vi "Fitness Tracker - Main.vi"() -> ()   [LabVIEW 2021]
uses:
  Lab 5/Lab 5 Code/Heading_TDef.ctl
  Main - States_SubVI.ctl
  <vilib>/Platform/TimedLoop/XDataNode/timing_clust.ctl
  <vilib>/Platform/TimedLoop/XDataNode/nitl_modes.ctl
  <vilib>/Platform/TimedLoop/XDataNode/wakeup.ctl
  ProducerConsumer Data Cluster_TDef.ctl
  Measurement Data Cluster_TDef.ctl
  <vilib>/myRIO/Instrument Drivers/Onboard IO/I2C/typedefs/I2C User Configuration.ctl
  <vilib>/myRIO/Instrument Drivers/Onboard IO/I2C/typedefs/I2C Transfer Rate.ctl
  <vilib>/myRIO/Instrument Drivers/Onboard IO/I2C/typedefs/I2C Reference.ctl
  <vilib>/myRIO/Common/Instrument Driver Framework/Utilities/typedefs/myRIO Generic Hardware Reference.ctl
  <vilib>/myRIO/Common/Instrument Driver Framework/Utilities/typedefs/Hardware Version Enum.ctl
  <vilib>/myRIO/Common/Instrument Driver Framework/Utilities/typedefs/myRIO v1.0 Reference.ctl
  <vilib>/myRIO/Common/Instrument Driver Framework/Utilities/typedefs/Generic FPGA Reference.ctl
  <vilib>/myRIO/Common/Instrument Driver Framework/myRIO v1.0/I2C/typedefs/I2C Channels Enum.ctl
  <vilib>/myRIO/Instrument Drivers/Onboard IO/I2C/typedefs/I2C Configuration.ctl
  <vilib>/userDefined/High Color/nirio_resource_hc.ctl
  <vilib>/myRIO/Common/Instrument Driver Framework/Utilities/vis/Is FPGA Ref Available.vi
  <vilib>/myRIO/Common/Instrument Driver Framework/myRIO v1.0/I2C/vis/myRIO v1.1 Open I2C.vi
  <vilib>/myRIO/Instrument Drivers/Onboard IO/I2C/vis/Configure.vi
  <vilib>/myRIO/Common/Instrument Driver Framework/Utilities/vis/Validate Channels.vi
  <vilib>/myRIO/Common/Instrument Driver Framework/myRIO v1.0/I2C/vis/myRIO v1.0 Reserve I2C.vi
  <vilib>/myRIO/Common/Instrument Driver Framework/myRIO v1.0/I2C/vis/myRIO v1.0 Build MUX Configuration I2C.vi
  <vilib>/myRIO/Common/Instrument Driver Framework/myRIO v1.0/Resource Manager/vis/myRIO v1.0 Reserve Channel List.vi
  <vilib>/myRIO/Common/Instrument Driver Framework/myRIO v1.0/Resource Manager/vis/myRIO v1.0 Create Configuration List.vi
  <vilib>/myRIO/Common/Instrument Driver Framework/myRIO v1.0/Resource Manager/vis/myRIO v1.0 Reserve Channel.vi
  <vilib>/myRIO/Common/Instrument Driver Framework/myRIO v1.0/Resource Manager/vis/myRIO v1.0 Unreserve Channel.vi
  <vilib>/myRIO/Common/Instrument Driver Framework/myRIO v1.0/Resource Manager/vis/myRIO v1.0 Build Mutex Name.vi
  <vilib>/Utility/error.llb/Error Cluster From Error Code.vi
  <vilib>/myRIO/Common/Instrument Driver Framework/myRIO v1.0/DIO/vis/myRIO v1.0 Write DIO.vi
  <vilib>/Utility/VariantDataType/GetNumericInfo.vi
  <vilib>/myRIO/Common/Instrument Driver Framework/myRIO v1.0/myRIO v1.1 Open.vi
  <vilib>/myRIO/Common/Instrument Driver Framework/Utilities/vis/IO Manager.vi
  <vilib>/myRIO/Common/Instrument Driver Framework/Utilities/vis/Configuration Manager.vi
  <vilib>/myRIO/Common/Instrument Driver Framework/myRIO v1.0/Resource Manager/vis/myRIO v1.0 Configure IO.vi
  <vilib>/myRIO/Common/Instrument Driver Framework/myRIO v1.0/myRIO v1.0 Close.vi
  <vilib>/myRIO/Common/Instrument Driver Framework/myRIO v1.0/I2C/vis/myRIO v1.0 Configure I2C.vi
  <vilib>/myRIO/Common/Instrument Driver Framework/myRIO v1.0/I2C/vis/myRIO v1.0 Write I2C.vi
  <vilib>/platform/TimedLoop/XDataNode/XDataNode.xnode
  <vilib>/myRIO/Express VI/Onboard IO/I2C/I2C Express VI.xnode
  <vilib>/myRIO/Instrument Drivers/Onboard IO/I2C/vis/myRIO I2C Open.xnode
  <vilib>/Platform/TimedLoop/XDataNode/XDNodeRunTimeDep.lvlib
  <vilib>/myRIO/Instrument Drivers/Onboard IO/DIO/DIO.lvlib
  <vilib>/myRIO/Instrument Drivers/Onboard IO/AI/AI.lvlib
  <vilib>/myRIO/Instrument Drivers/Onboard IO/I2C/I2C.lvlib
panel:
  out "x > y?":bool
  out "Gyro Rotation Out (degrees)":dbl[](array[numeric])
  out "element":dbl
  out "error out 4":errorcluster
  in  "error in (no error) 2":errorcluster
  out "error out 3":errorcluster
  out "Loop 2 Time":i32
  out "GNRMC String Array":string[](array[string])
  out "Step Counter Map":T1(graph)
  out "Producer Loop Time (ms)":i32
  out "Consumer Loop Time (ms)":i32
  out "Heart Rate":dbl
  out "Latitude N (deg)":dbl
  out "DIP State":T2
  out "Time Elapsed (min)":dbl
  out "error out 2":errorcluster caption="error out"
  out "North":dbl
  out "East":dbl
  out "Heading String 2":T3
  out "Heading":dbl
  out "Steps":i32
  in  "error in (no error)":errorcluster
  in  "Reset Gyro":bool
  out "Acceleration (g)":T4(graph)
  out "Velocity":T5(graph)
  out "Rotation":T4(graph)
  out "Acceleration (ms^2)":dbl[](array[numeric])
  out "Velocity Cluster Out":cluster{i16, i16, i16}
  out "Rotation Cluster Out":T6
  out "error out":errorcluster
  in  "stop":bool
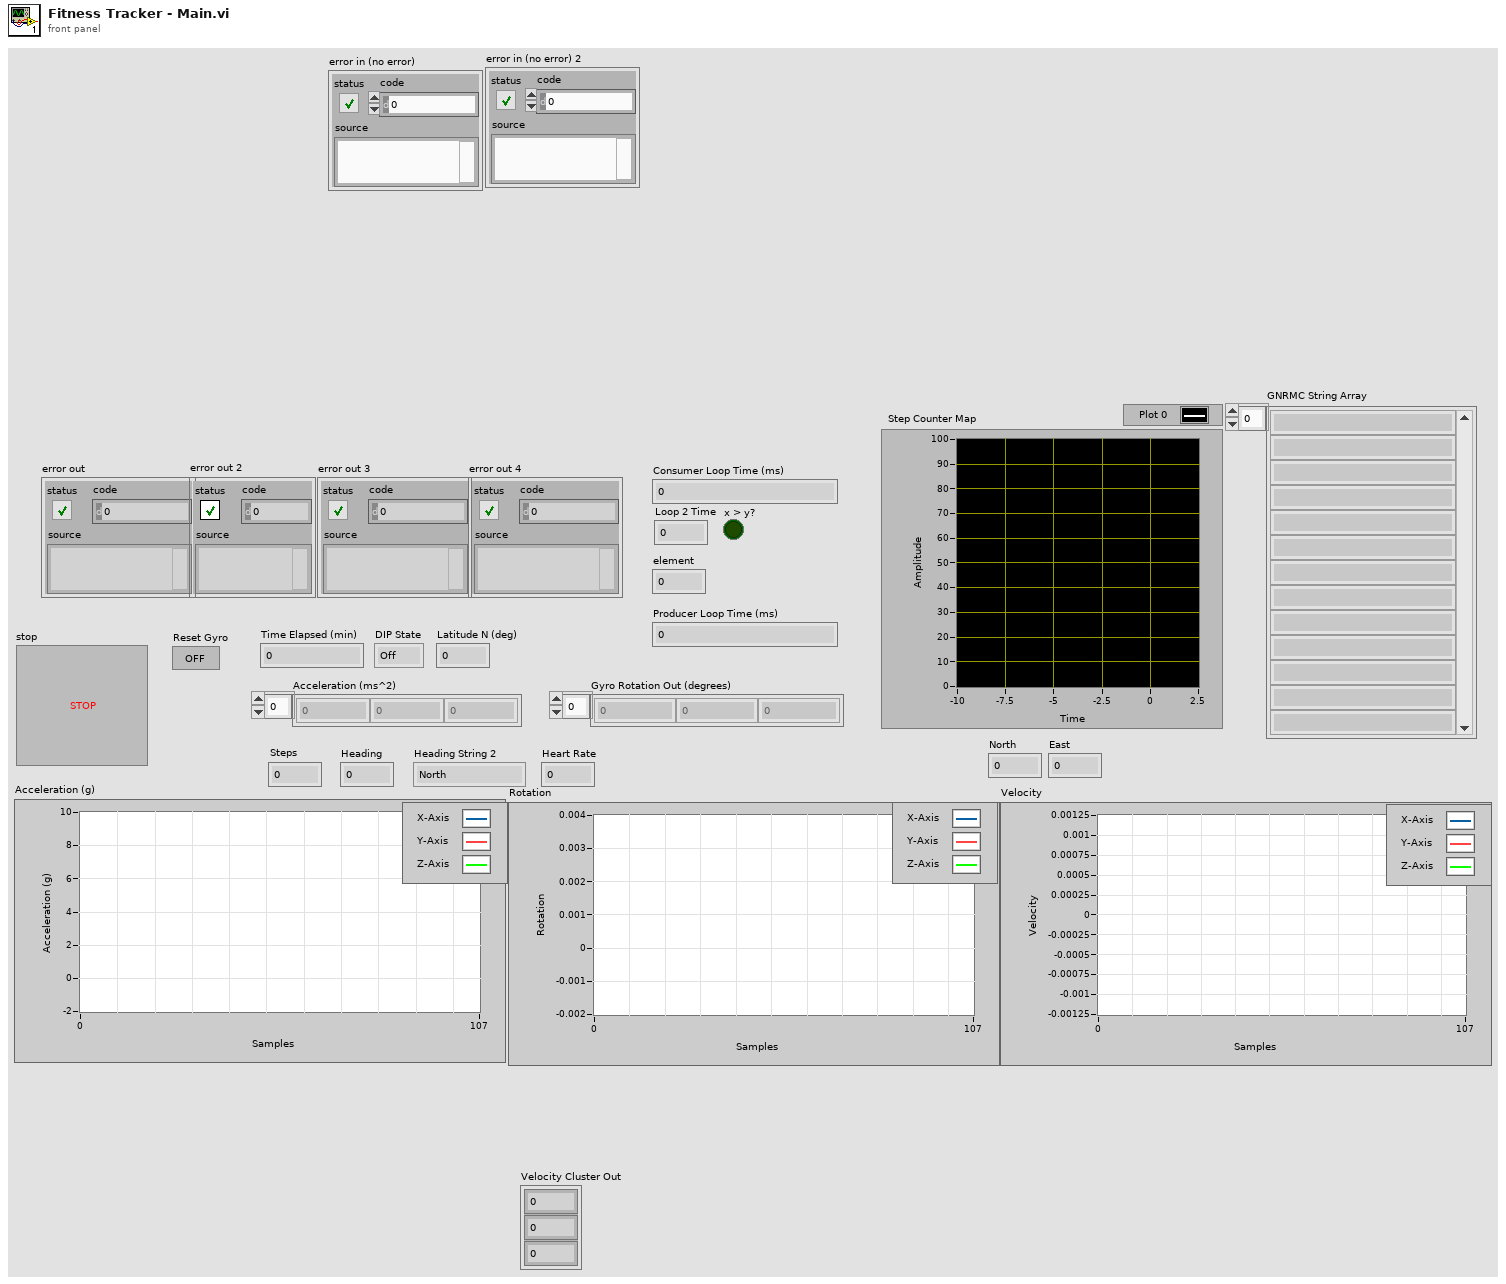
[diagram p1: front panel]
types:
  T1 = cluster{"X Displacement Array ":dbl[], "Y Displacement Array ":dbl[]}
  T2 = typedef "Main - States_SubVI.ctl" = enum16{"Off", "Record", "Upload", "Shutdown", "Error"}
  T3 = typedef "Heading_TDef.ctl" = enum16{"North ", "North East", "East", "Southeast", "South", "Southwest", "West", "Northwest"}
  T4 = cluster{"X-Axis":dbl, "Y-Axis":dbl, "Z-Axis":dbl}
  T5 = cluster{"Velocity":dbl, "Velocity":dbl, "Velocity":dbl}
  T6 = cluster{"integral x(t)":dbl, "integral x(t)":dbl, "integral x(t)":dbl}
  T7 = typedef "Measurement Data Cluster_TDef.ctl" = cluster{"Step Count":i32, "East Displacement":dbl, "North Displacement":dbl, "Longitude":dbl, "Latitude":dbl, "Heart Rate":dbl, "Time Elapsed (min)":dbl}
  T8 = typedef "ProducerConsumer Data Cluster_TDef.ctl" = cluster{"Accelerometer":dbl[], "Gyro":dbl[], "Magnetometer":dbl, "Time":i32, "Pulse":dbl}
  T9 = typedef "DIO.lvlib/DIO Reference.ctl" = cluster{"myRIO Reference":T10, "DIO Channels List":T14}
  T10 = typedef "myRIO Generic Hardware Reference.ctl" = cluster{"myRIO Model":T11, "myRIO Hardware Reference":T12}
  T11 = typedef "Hardware Version Enum.ctl" = enum16{"Unknown", "myRIO-1900", "myRIO-1950", "roboRIO", "NI ELVIS RIO CM", "ELVIS III"}
  T12 = typedef "myRIO v1.0 Reference.ctl" = cluster{"Generic FPGA Reference":T13, "Allow multiple opens":bool}
  T13 = typedef "Generic FPGA Reference.ctl" = refnum<k20>
  T14 = typedef "DIO Channels List.ctl" = T15[]
  T15 = typedef "DIO Channels Enum.ctl" = enum16{"Not Connected", "C/DIO0", "C/DIO1", "C/DIO2", "C/DIO3", "C/DIO4", "C/DIO5", "C/DIO6", "C/DIO7", "A/DIO0", "A/DIO1", "A/DIO2", "A/DIO3", "A/DIO4", "A/DIO5", "A/DIO6", "A/DIO7", "A/DIO8", "A/DIO9", "A/DIO10", "A/DIO11", "A/DIO12", "A/DIO13", "A/DIO14", "A/DIO15", "A/DIO16", "A/DIO17", "A/DIO18", "A/DIO19", "B/DIO0", "B/DIO1", "B/DIO2", "B/DIO3", "B/DIO4", "B/DIO5", "B/DIO6", "B/DIO7", "B/DIO8", "B/DIO9", "B/DIO10", "B/DIO11", "B/DIO12", "B/DIO13", "B/DIO14", "B/DIO15", "B/DIO16", "B/DIO17", "B/DIO18", "B/DIO19", "LED0", "LED1", "LED2", "LED3", "Button0", "DIO/DIO0", "DIO/DIO1", "DIO/DIO2", "DIO/DIO3", "DIO/DIO4", "DIO/DIO5", "DIO/DIO6", "DIO/DIO7", "DIO/DIO8", "DIO/DIO9", "SPI/CS0", "SPI/CS1", "SPI/CS2", "SPI/CS3", "LED RADIO (Green)", "LED RADIO (Red)", "LED COMM (Green)", "LED COMM (Red)", "LED MODE (Green)", "LED MODE (Red)"}
  T16 = typedef "XDNodeRunTimeDep.lvlib/timing_clust.ctl" = cluster{"Expected End [f-1]":u64, "Actual End [f-1]":u64, "Finished Late? [f-1]":bool, "Expected End [i-1]":u64, "Actual End [i-1]":u64, "Finished Late? [i-1]":bool, "Expected Start [i]":u64, "Actual Start [i]":u64, "Expected Start [f]":u64, "Actual Start [f]":u64, "Source Name":string, "Structure Name":string, "Period":i64, "Deadline":i64, "Offset":i64, "Start":i64, "Priority":i32, "Timeout":i32, "Mode":T17, "Wakeup Reason":T18, "Error":errorcluster, "Source Type":string, "Secondary Source Type":string, "Global End Time":u64, "Global Start Time":u64, "Frame Duration":u64, "Iteration Duration":u64, "Assigned CPU":i32, "I/O Scan Engine Mode":u32}
  T17 = typedef "XDNodeRunTimeDep.lvlib/nitl_modes.ctl" = enum32{"No Change", "Process missed periods, maintain original phase", "Discard missed periods, maintain original phase", "Process missed periods, ignore original phase", "Discard missed periods, ignore original phase"}
  T18 = typedef "XDNodeRunTimeDep.lvlib/wakeup.ctl" = enum32{"Normal", "Aborted", "Asynchronous wakeup", "Timing source error", "Timed loop error", "Timeout"}
  T19 = typedef "I2C.lvlib/I2C Reference.ctl" = cluster{"myRIO Reference":T10, "I2C Channels Enum":T20, "I2C Configuration":T21}
  T20 = typedef "I2C Channels Enum.ctl" = enum16{"Not Connected", "A/I2C", "B/I2C", "I2C/I2C"}
  T21 = typedef "I2C.lvlib/I2C Configuration.ctl" = cluster{"I2C Transfer Rate":T22}
  T22 = typedef "I2C.lvlib/I2C Transfer Rate.ctl" = enum16{"Standard mode (100 kbps)", "Fast mode (400 kbps)"}
  T23 = typedef "AI.lvlib/AI Reference.ctl" = cluster{"myRIO Reference":T10, "AI Channels List":T24, "AI Scaling Constants List":T26}
  T24 = typedef "AI Channels List.ctl" = T25[]
  T25 = typedef "AI Channels Enum.ctl" = enum16{"Not Connected", "AudioIn/Left", "AudioIn/Right", "C/AI0", "C/AI1", "A/AI0", "A/AI1", "A/AI2", "A/AI3", "A/AI4", "A/AI5", "A/AI6", "A/AI7", "B/AI0", "B/AI1", "B/AI2", "B/AI3", "B/AI4", "B/AI5", "B/AI6", "B/AI7", "AI/AI0", "AI/AI1", "AI/AI2", "AI/AI3", "A/AI0 (DIFF)", "A/AI1 (DIFF)", "A/AI2 (DIFF)", "A/AI3 (DIFF)", "B/AI0 (DIFF)", "B/AI1 (DIFF)", "B/AI2 (DIFF)", "B/AI3 (DIFF)"}
  T26 = typedef "Analog Scaling Constants List.ctl" = T27[]
  T27 = typedef "Analog Scaling Constants.ctl" = cluster{"LSB Weight (Volts)":dbl, "Offset (Volts)":dbl, "Signed?":bool}
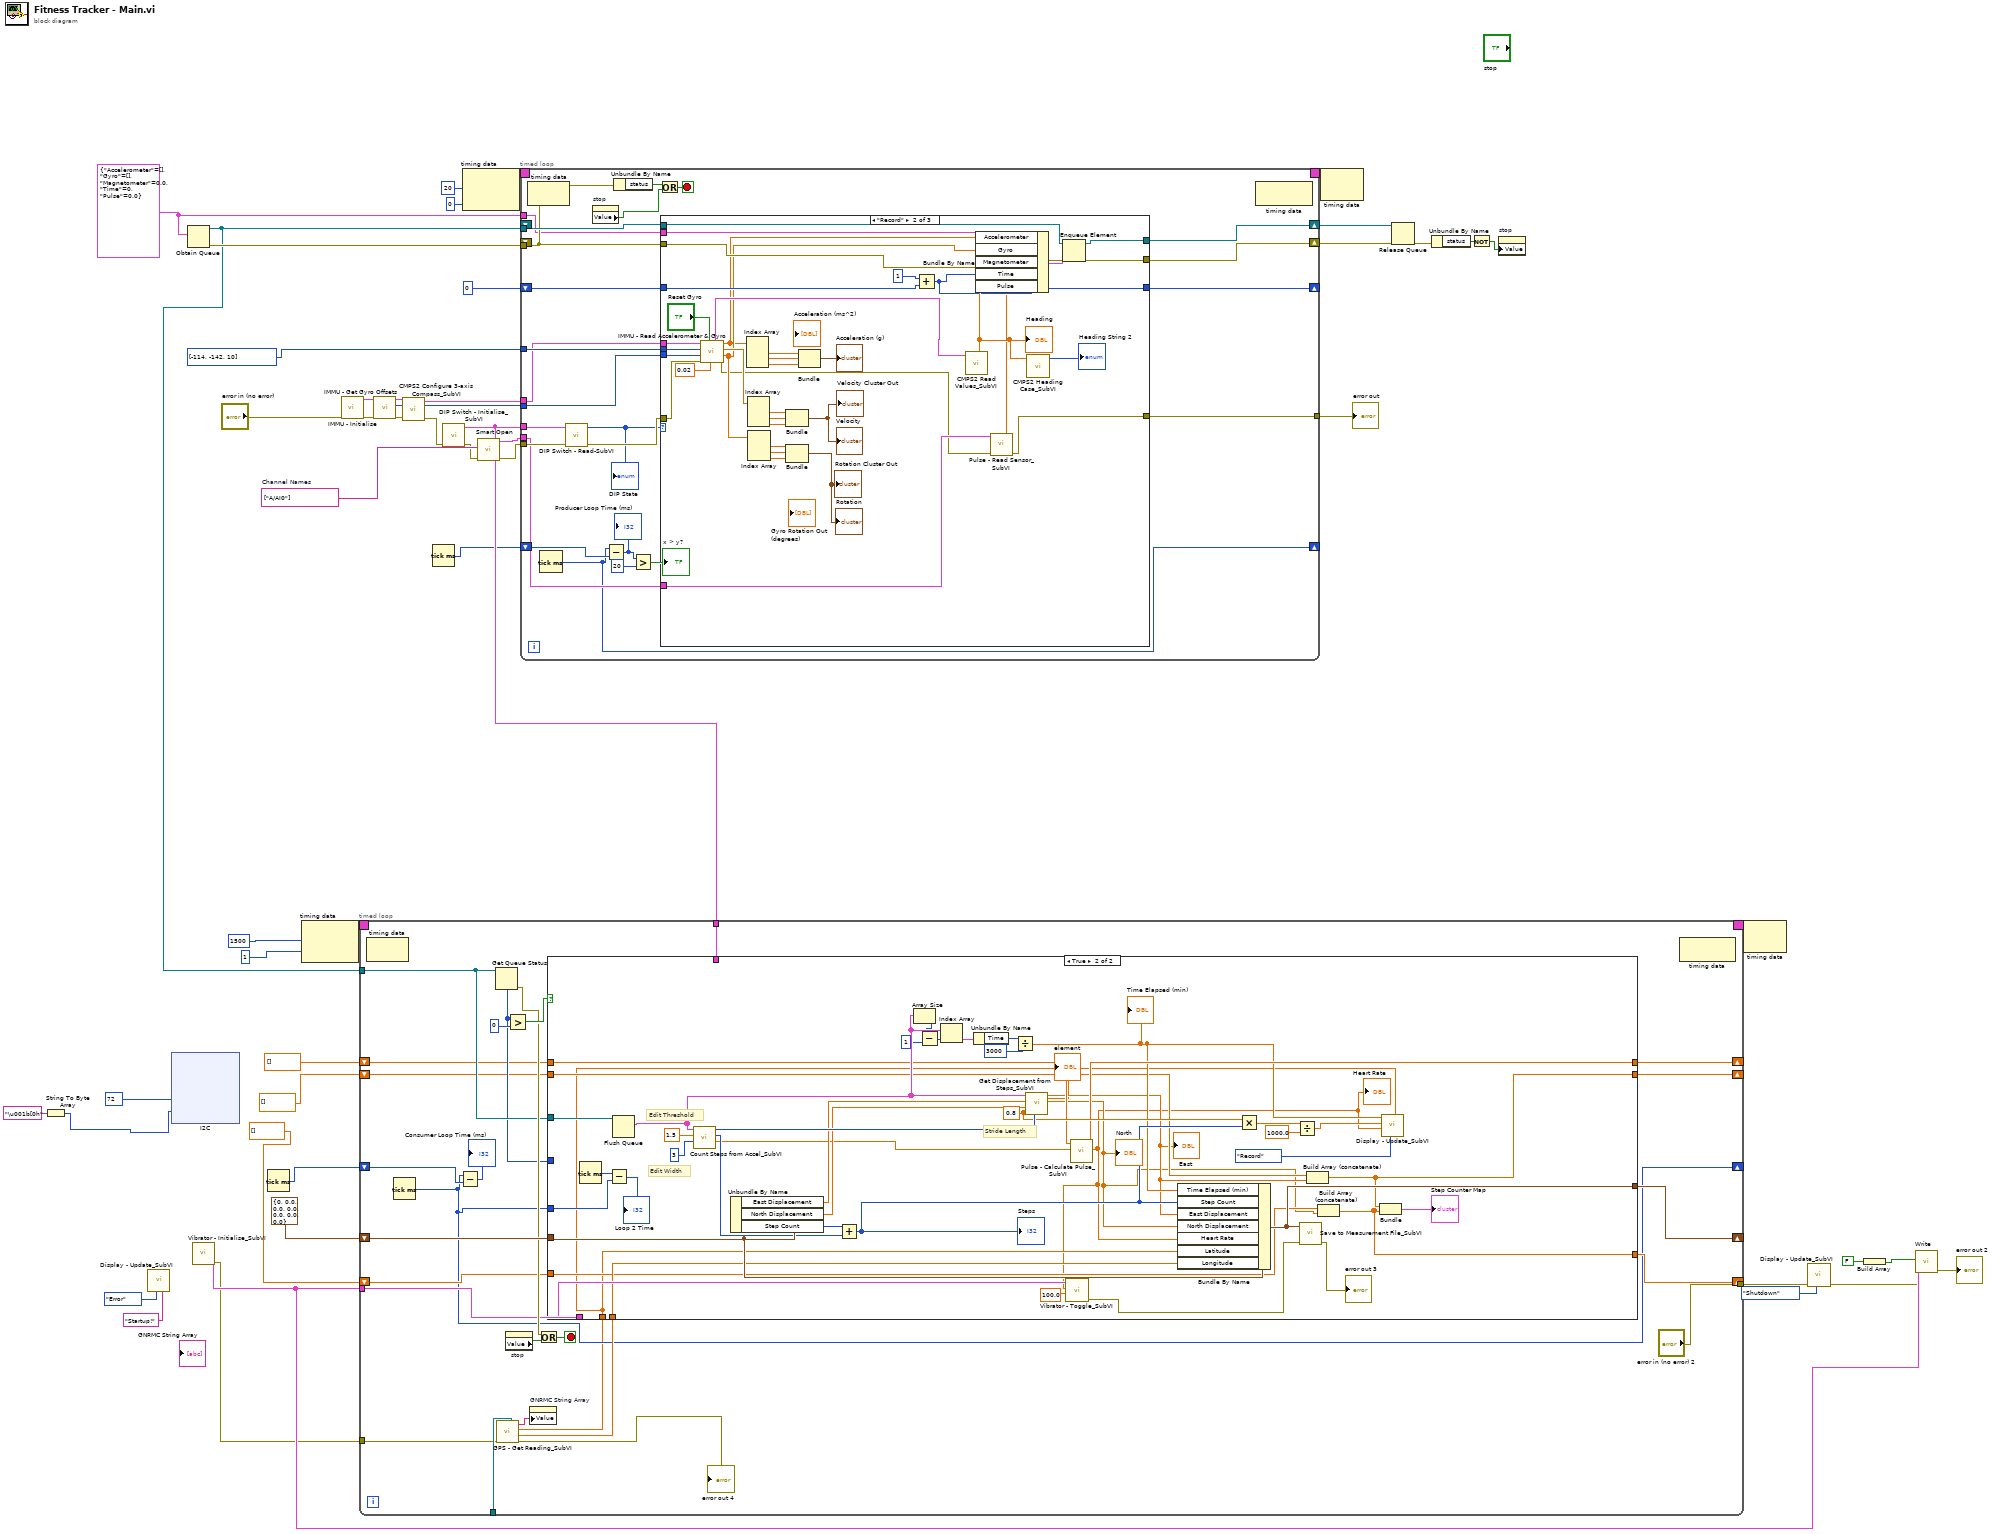
[diagram p0: block diagram]
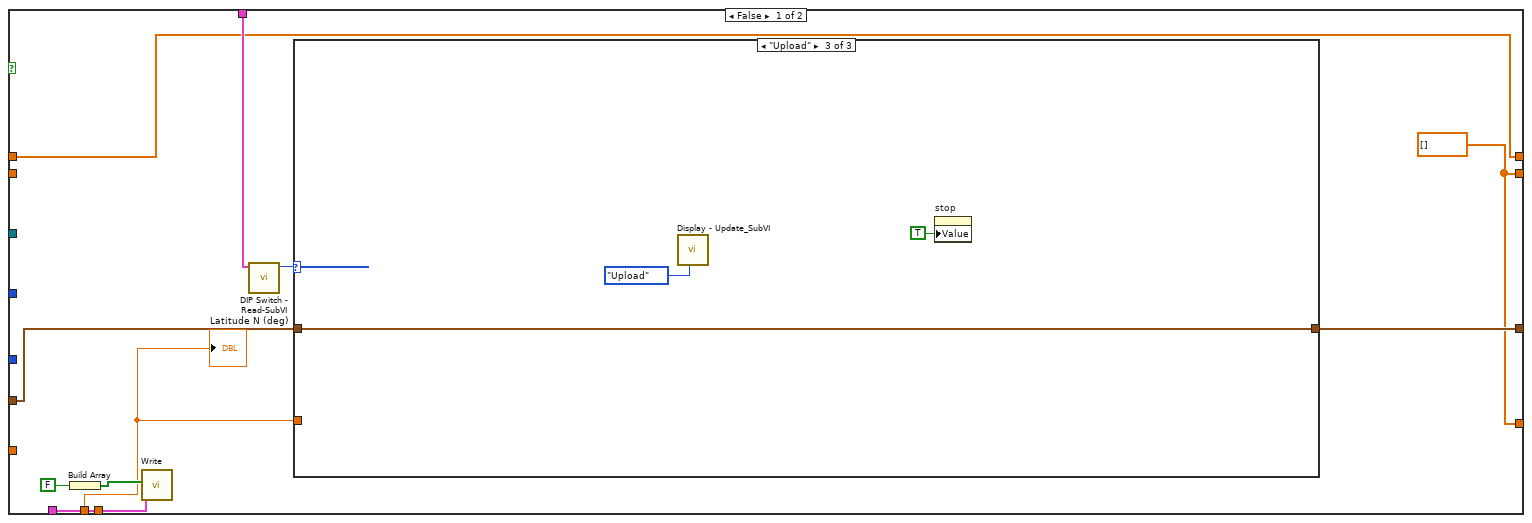
[diagram p2: hidden frame]
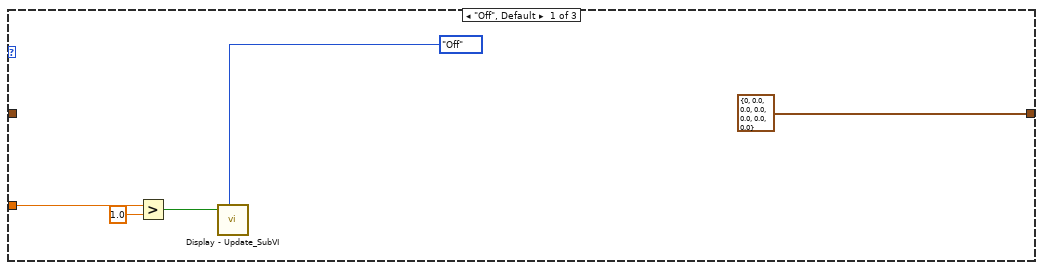
[diagram p3: hidden frame]
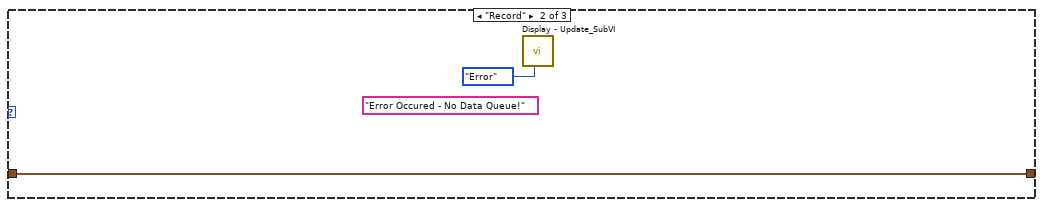
[diagram p4: hidden frame]
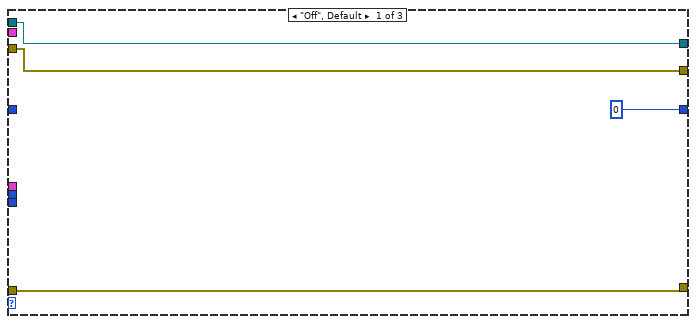
[diagram p5: hidden frame]
diagram:
  w22 = tag[] ["A/AI0"]  # Channel Names
  w28 = T8 {"Accelerometer"=[], "Gyro"=[], "Magnetometer"=0.0, "Time"=0, "Pulse"=0.0}
  n1 = String To Byte Array(string="\u001b[0h") -> (unsigned byte array=w7:u8[])
  n2 = call "Display - Update_SubVI.vi"("Error Msg In"="Startup!", "Enum"=Main_-_States_SubVI."Error") -> ()  [unwired: 9 in, 1 out]
  n3 = xnode "I2C"("Slave Address (7-bit)"=72, "Bytes to Write"=w7) -> ()  [unwired: 1 in, 1 out]
  n4 = Obtain Queue(element data type=w28) -> (queue out=w43:refnum<queue>, error out=w44:errorcluster)  [unwired: 4 in, 1 out]
  n5 = call "Vibrator - Initialise_SubVI.vi"() -> ("error out"=w1:errorcluster, "DIO Ref Out"=w13:T9)  [unwired: 10 in]
  n6 = Tick Count (ms)() -> (millisecond timer value=w18:u32)
  n7 = node-c288(i64 1500 ("Period"), 1 ("Processor")) -> (w49:T16)
  n8 = call "IMMU - Initialise.vi"("error in (no error)"="error in (no error)") -> ("error out"=w38:errorcluster, "I2C Ref Out"=w37:T19)  [unwired: 9 in]
  n9 = call "IMMU - Get Gyro Offsets.vi"("error in (no error)"=w38, "I2C Ref In"=w37) -> ("error out"=w30:errorcluster, "Output Offset Array (int)"=w35:i16[], "I2C Ref Out"=w31:T19)  [unwired: 7 in]
  n10 = call "CMPS2 Configure 3-axis Compass_SubVI.vi"("error in (no error)"=w30, "I2C Ref In"=w31) -> ("error out"=w25:errorcluster, "I2C Ref Out"=w29:T19)  [unwired: 8 in]
  n11 = Tick Count (ms)() -> (millisecond timer value=w10:u32)
  n12 = call "DIP Switch - Initialise_SubVI.vi"("error in (no error)"=w25) -> ("error out"=w21:errorcluster, "AI Ref Out"=w24:T23)  [unwired: 9 in]
  n13 = timed-loop {
    timing: w49 -> [_]
    timing-out: [_] -> w48
    tunnel: w43 -> [w72]
    shift-right: [w71] -> _
    shift-left: T7 {"Step Count"=0, "East Displacement"=0.0, "North Displacement"=0.0, "Longitude"=0.0, "Latitude"=0.0, "Heart Rate"=0.0, "Time Elapsed (min)"=0.0} -> [w74]
    tunnel: w24 -> [w70]
    tunnel: w13 -> [w69]
    shift-right: [w58] -> _
    shift-left: w18 -> [w66]
    shift-right: [w64] -> _
    shift-left: dbl[] [] ("threshold") -> [w65]
    shift-right: [w59] -> _
    shift-left: dbl[] [] ("threshold") -> [w61]
    shift-right: [w60] -> _
    shift-left: dbl[] [] ("threshold") -> [w62]
    tunnel: ["error in (no error) 2"] -> w2
    tunnel: [w53] -> _
    tunnel: w1 -> [w52]
    stop <- w77 stop-if-true
    n14 = node-c288() -> ()  [unwired: 1 in, 1 out]
    n15 = Tick Count (ms)() -> (millisecond timer value=w58:u32)
    n16 = Subtract(x=w58, y=w66) -> (x-y=→"Consumer Loop Time (ms)":u32)
    n17 = Get Queue Status(queue=w72) -> (error out=w73:errorcluster, # elements in queue=w68:i32)  [unwired: 2 in, 6 out]
    n18 = call "GPS - Get Reading_SubVI.vi"("error in (no error) 2"=w52) -> ("error out"=→"error out 4":errorcluster, "Longitude W (deg)"=w63:dbl, "Latitude N (deg)"=w56:dbl, "GNRMC String Array"=w55:string[], "VISA resource name out"=w53:refnum<visa-resource-name>)  [unwired: 6 in]
    n19 = property on="stop" class="Bool (strict)"() -> ("Value"=w76:bool)  [unwired: 2 in, 2 out]
    n20 = Greater?(x=w68, y=0) -> (0:w75:bool)
    n21 = property on="GNRMC String Array" class="Arr (strict)"("Value"=w55) -> ()  [unwired: 2 in, 2 out]
    n22 = Or(x=w73, y=w76) -> (x .or. y?=w77:bool)
    n23 = case shown="True" w75 {
      tunnel: w74 -> [w87 w139]
      tunnel: [w88 w134] -> w71
      tunnel: w72 -> [_ w141]
      tunnel: w70 -> [w85 _]
      tunnel: w69 -> [w82 w121]
      tunnel: w68 -> [_ _]
      tunnel: w65 -> [w81 w119]
      tunnel: [w81 w118] -> w64
      tunnel: w56 -> [w80 w102]
      tunnel: w63 -> [_ w114]
      tunnel: w62 -> [_ w112]
      tunnel: w61 -> [_ w110]
      tunnel: [w79 w108] -> w60
      tunnel: [w79 w107] -> w59
      tunnel: w58 -> [_ w105]
      frame False {
        w79 = dbl[] [] ("threshold")
        n24 = Build Array(FALSE) -> (w84:bool[])
        n25 = call <vilib>:"Write.vi"("Values"=w84, "DIO Ref In"=w82) -> ()  [unwired: 7 in, 2 out]
        n26 = call "DIP Switch - Read-SubVI.vi"("AI Ref In"=w85) -> ("DIP State"=w86:T2)  [unwired: 9 in, 1 out]
        n27 = case shown="\"Upload\"" w86 {
          tunnel: [T7 {"Step Count"=0, "East Displacement"=0.0, "North Displacement"=0.0, "Longitude"=0.0, "Latitude"=0.0, "Heart Rate"=0.0, "Time Elapsed (min)"=0.0} w95 w98] -> w88
          tunnel: w87 -> [_ w95 w98]
          tunnel: w80 -> [w89 _ _]
          frame "Off", Default {
            n28 = Greater?(x=w89, y=1.0) -> (0:w91:bool)
            n29 = call "Display - Update_SubVI.vi"("Enum"=Main_-_States_SubVI."Off", "GPS Connected?"=w91) -> ()  [unwired: 9 in, 1 out]
          }
          frame "Record" {
            (unwired) "Error Occured - No Data Queue!" ("Error Msg In")
            n30 = call "Display - Update_SubVI.vi"("Enum"=Main_-_States_SubVI."Error") -> ()  [unwired: 10 in, 1 out]
          }
          frame "Upload" {
            n31 = call "Display - Update_SubVI.vi"("Enum"=Main_-_States_SubVI."Upload") -> ()  [unwired: 10 in, 1 out]
            n32 = property on="stop" class="Bool (strict)"("Value"=TRUE ("stop")) -> ()  [unwired: 2 in, 2 out]
          }
        }
        "Latitude N (deg)" <- w80
      }
      frame True {
        w124 = 0.8 ("Stride Length")
        # "Stride Length"
        # "Edit Width"
        # "Edit Threshold"
        n33 = Tick Count (ms)() -> (millisecond timer value=w104:u32)
        n34 = Subtract(x=w104, y=w105) -> (x-y=→"Loop 2 Time":u32)
        n35 = Flush Queue(queue=w141) -> (remaining elements=w128:T8[])  [unwired: 1 in, 2 out]
        n36 = call "Count Steps from Accel_SubVI.vi"("width"=3, "threshold"=1.5, "Queue Elements In"=w128) -> ("Pulse Array"=w120:dbl[], "Step Count"=w137:i32, "Step Indices"=w138:i32[])  [unwired: 6 in]
        n37 = Unbundle By Name(w139) -> ("East Displacement"=w136:dbl, "North Displacement"=w135:dbl, "Step Count"=w140:i32)
        n38 = Add(x=w140, y=w137) -> (x+y=w132:i32)
        "Steps" <- w132
        n39 = Array Size(array=w128) -> (size(s)=w126:i32)
        n40 = Subtract(x=w126, y=1) -> (x-y=w127:i32)
        n41 = Index Array(array=w128, index=w127) -> (element=w131:T8)
        n42 = Unbundle By Name(w131) -> ("Time"=w130:i32)
        n43 = Divide(x=w130, y=3000) -> (x/y=w113:dbl)
        "Time Elapsed (min)" <- w113
        n44 = call "Get Displacement from Steps_SubVI.vi"("Step Indices"=w138, "Stride Length"=w124, "North Displacement In"=w135, "East Displacement In"=w136, "Queue Elements In"=w128) -> ("North Displacement Out"=w109:dbl, "East Displacement Out"=w111:dbl, "element"=→"element":dbl)  [unwired: 4 in]
        "East" <- w111
        "North" <- w109
        n45 = call "Pulse - Calculate Pulse_SubVI.vi"("New Pulse Data"=w120, "Existing Pulse Data"=w119) -> ("Heart Rate"=w101:dbl, "Pulse Array Out"=w118:dbl[])  [unwired: 7 in, 1 out]
        "Heart Rate" <- w101
        n46 = call "Vibrator - Toggle_SubVI.vi"("Max Pulse Threshold"=100.0, "Pulse In"=w101, "DIO Ref Out"=w121) -> ("error out"=w116:errorcluster)  [unwired: 8 in]
        n47 = Bundle By Name(cluster=w139, "Time Elapsed (min)"=w113, "Step Count"=w132, "East Displacement"=w111, "North Displacement"=w109, "Heart Rate"=w101, "Latitude"=w102, "Longitude"=w114) -> (w134:T7)
        n48 = Multiply(x=w124, y=w132) -> (x*y=w123:dbl)
        n49 = Divide(x=w123, y=1000.0) -> (x/y=w103:dbl)
        n50 = call "Save to Measurement File_SubVI.vi"("error in (no error)"=w116, "Input Cluster Data"=w134) -> ("error out"=→"error out 3":errorcluster)  [unwired: 9 in]
        n51 = Build Array (concatenate)(w112, w111) -> (w108:dbl[])
        n52 = Build Array (concatenate)(w110, w109) -> (w107:dbl[])
        n53 = Bundle(w108, w107) -> (→"Step Counter Map":cluster{dbl[], dbl[]})  [unwired: 1 in]
        n54 = call "Display - Update_SubVI.vi"("Lat"=w102, "Enum"=Main_-_States_SubVI."Record", "Heart Rate"=w101, "Distance Run"=w103, "Time Elapsed"=w113) -> ()  [unwired: 6 in, 1 out]
      }
    }
    n55 = node-c288() -> ()  [unwired: 1 in, 1 out]
  }
  n56 = node-c288(i64 20 ("Period"), 0 ("Processor")) -> (w51:T16)
  n57 = call <vilib>:"Smart Open.vi"("error in (no error)"=w21, "Channel Names"=w22) -> ("error out"=w20:errorcluster, "AI Ref Out"=w19:T23)  [unwired: 8 in]
  n58 = timed-loop {
    timing: w51 -> [_]
    timing-out: [_] -> w50
    tunnel: w43 -> [w163]
    tunnel: w44 -> [w162]
    shift-right: [w164] -> w42
    shift-left: _ -> [_]
    shift-right: [w161] -> w41
    shift-left: _ -> [_]
    tunnel: i16[] [-114, -142, 10] ("Accel Offset Array In") -> [w166]
    tunnel: w35 -> [w165]
    tunnel: w20 -> [w156]
    tunnel: w29 -> [w160]
    tunnel: w28 -> [w159]
    shift-right: [w157] -> _
    shift-left: 0 -> [w158]
    tunnel: w24 -> [w154]
    tunnel: [w152] -> w23
    tunnel: w19 -> [w151]
    shift-right: [w149] -> _
    shift-left: w10 -> [w150]
    stop <- w169 stop-if-true
    n59 = node-c288() -> ()  [unwired: 1 in, 1 out]
    n60 = Tick Count (ms)() -> (millisecond timer value=w149:u32)
    n61 = call "DIP Switch - Read-SubVI.vi"("error in (no error)"=w156, "AI Ref In"=w154) -> ("error out"=w155:errorcluster, "DIP State"=w153:T2)  [unwired: 8 in]
    "DIP State" <- w153
    n62 = property on="stop" class="Bool (strict)"() -> ("Value"=w167:bool)  [unwired: 2 in, 2 out]
    n63 = Subtract(x=w149, y=w150) -> (x-y=w148:u32)
    "Producer Loop Time (ms)" <- w148
    n64 = Unbundle By Name(w162) -> ("status"=w168:bool)
    n65 = Greater?(x=w148, y=u32 20) -> (0:→"x > y?":bool)
    n66 = Or(x=w168, y=w167) -> (x .or. y?=w169:bool)
    n67 = case shown="\"Record\"" w153 {
      tunnel: w166 -> [_ w206 _]
      tunnel: w165 -> [_ w205 _]
      tunnel: [w172 w198 w213] -> w164
      tunnel: w163 -> [w173 w197 w214]
      tunnel: w162 -> [w172 w196 w213]
      tunnel: [w173 w194 w214] -> w161
      tunnel: w155 -> [w170 w192 w211]
      tunnel: w160 -> [_ w191 _]
      tunnel: w159 -> [_ w189 _]
      tunnel: w158 -> [_ w185 w212]
      tunnel: [0 w184 w212] -> w157
      tunnel: [w170 w183 w211] -> w152
      tunnel: w151 -> [_ w181 _]
      frame "Off", Default {
      }
      frame "Record" {
        n68 = call "IMMU - Read Accelerometer & Gyro.vi"("dt"=0.02, "Reset Gyro"="Reset Gyro", "error in (no error)"=w192, "Gyro Offset Array In"=w205, "Accel Offset Array In"=w206, "I2C Ref In"=w191) -> ("error out"=w178:errorcluster, "Gyro Rotation Out (degrees)"=w180:dbl[], "Gyro Rotational Velocity Out (deg/s)"=w188:dbl[], "Output Acceleration Array (ms^2)"=w179:dbl[], "I2C Ref Out"=w193:T19)  [unwired: 1 in]
        n69 = Index Array(array=w179) -> (element #1=w204:dbl, element #2=w203:dbl, element #3=w202:dbl)  [unwired: 3 in]
        n70 = Index Array(array=w188) -> (element #1=w201:dbl, element #2=w200:dbl, element #3=w199:dbl)  [unwired: 3 in]
        n71 = Index Array(array=w180) -> (element #1=w210:dbl, element #2=w209:dbl, element #3=w208:dbl)  [unwired: 3 in]
        n72 = Bundle(w201, w200, w199) -> (→"Velocity Cluster Out" →"Velocity":cluster{dbl, dbl, dbl})  [unwired: 1 in]
        n73 = Bundle("integral x(t)"=w210, "integral x(t)"=w209, "integral x(t)"=w208) -> (→"Rotation Cluster Out" →"Rotation":T6)  [unwired: 1 in]
        n74 = Bundle(w204, w203, w202) -> (→"Acceleration (g)":cluster{dbl, dbl, dbl})  [unwired: 1 in]
        n75 = Add(x=1, y=w185) -> (x+y=w184:i32)
        n76 = call "CMPS2 Read Values_SubVI.vi"("I2C Ref In"=w193) -> ("Heading"=w187:dbl)  [unwired: 5 in, 5 out]
        "Heading" <- w187
        n77 = call "Pulse - Read Sensor_SubVI.vi"("error in (no error)"=w178, "AI Ref In"=w181) -> ("error out"=w183:errorcluster, "Pulse Sensor Read Out"=w182:dbl)  [unwired: 8 in]
        n78 = Bundle By Name(cluster=w189, "Accelerometer"=w179, "Gyro"=w180, "Magnetometer"=w187, "Time"=w184, "Pulse"=w182) -> (w190:T8)
        n79 = call "CMPS2 Heading Case_SubVI.vi"("Numeric"=w187) -> ("Heading String 2"=→"Heading String 2":T3)  [unwired: 10 in]
        n80 = Enqueue Element(queue=w197, element=w190, error in (no error)=w196) -> (queue out=w194:refnum<queue>, error out=w198:errorcluster)  [unwired: 1 in, 1 out]
      }
      frame "Upload" {
      }
    }
    n81 = node-c288() -> ()  [unwired: 1 in, 1 out]
  }
  "error out" <- w23
  n82 = node-c288(w50) -> ()  [unwired: 1 out]
  n83 = Release Queue(queue=w41, error in (no error)=w42) -> (error out=w34:errorcluster)  [unwired: 1 in, 2 out]
  n84 = Unbundle By Name(w34) -> ("status"=w33:bool)
  n85 = Not(x=w33) -> (.not. x?=w32:bool)
  n86 = property on="stop" class="Bool (strict)"("Value"=w32) -> ()  [unwired: 2 in, 2 out]
  n87 = node-c288(w48) -> ()  [unwired: 1 out]
  n88 = call "Display - Update_SubVI.vi"("Enum"=Main_-_States_SubVI."Shutdown", "error in (no error)"=w2) -> ("error out"=w12:errorcluster)  [unwired: 9 in]
  n89 = Build Array(FALSE) -> (w15:bool[])
  n90 = call <vilib>:"Write.vi"("error in (no error)"=w12, "Values"=w15, "DIO Ref In"=w13) -> ("error out"=→"error out 2":errorcluster)  [unwired: 6 in, 1 out]
